vi "emi_Wait for loops to stop.vi"(0 "Loop exlusion[0,..]":u16[](array[numeric])=[0], 7 "Timeout ms(5000)":i32=5000, 11 "error in (no error)":errorcluster) -> (15 "error out":errorcluster)   [LabVIEW 2011]
doc: "Wait for all indexed loops to close. Generates error if times out.\n\nRens regardless of error"
uses:
  Loop control/Private/_emi_Loop control int action.ctl
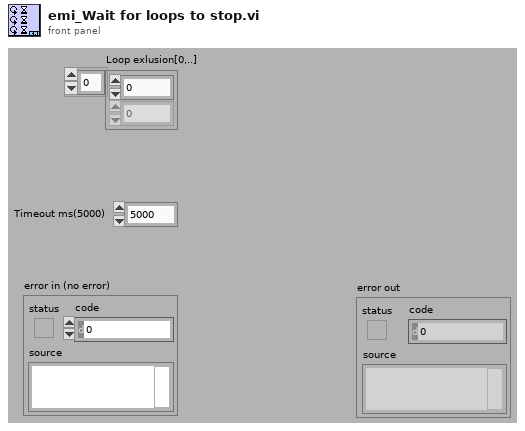
[diagram p1: front panel]
types:
  T1 = typedef "_emi_Loop control int action.ctl" = enum16{"Init index", "Get index", "Set index", "Get Size"}
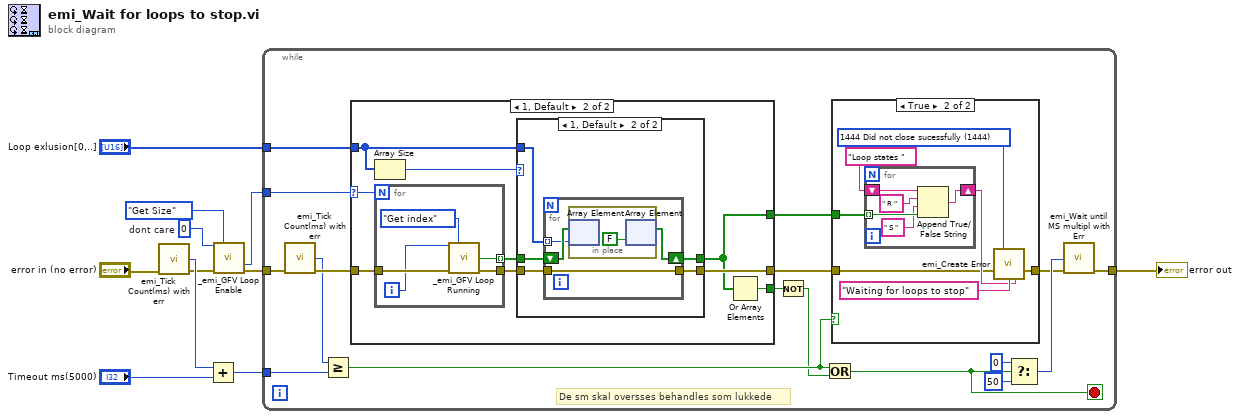
[diagram p0: block diagram]
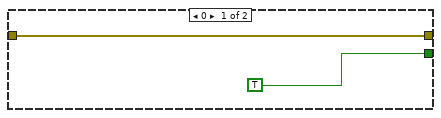
[diagram p3: hidden frame]
diagram:
  w1 = 0  # dont care
  n1 = call "emi_Tick Count(ms) with err.vi"("error in (no error)"="error in (no error)") -> ("millisecond timer value"=w7:u32, "error out"=w5:errorcluster)  [unwired: 13 in]
  n2 = Add(x=w7, y="Timeout ms(5000)") -> (x+y=w2:u32)
  n3 = call "_emi_GFV Loop Enable.vi"("Loop Index/Numb"=w1, "Action(Get Index)"=_emi_Loop_control_int_action."Get Size", "error in (no error)"=w5) -> ("Size"=w3:i32, "error out"=w4:errorcluster)  [unwired: 9 in, 2 out]
  n4 = while {
    tunnel: "Loop exlusion[0,..]" -> [w28]
    tunnel: [w27] -> w10
    tunnel: w4 -> [w22]
    tunnel: w3 -> [w23]
    tunnel: w2 -> [w20]
    stop <- w12 stop-if-true
    # "De sm skal oversses behandles som lukkede"
    n5 = call "emi_Tick Count(ms) with err.vi"("error in (no error)"=w22) -> ("millisecond timer value"=w19:u32, "error out"=w21:errorcluster)  [unwired: 13 in]
    n6 = Greater Or Equal?(x=w19, y=w20) -> (x >= y?=w15:bool)
    n7 = case shown="1, Default" w23 {
      selector: w23 -> [_ w51]
      tunnel: w21 -> [w43 w52]
      tunnel: w28 -> [_ w47]
      tunnel: [w43 w46] -> w18
      tunnel: [TRUE w44] -> w14
      tunnel: [_ w45] -> w17
      frame 0 {
      }
      frame 1, Default {
        n8 = Array Size(array=w47) -> (size(s)=w49:i32)
        n9 = for {
          N: w51 -> [_]
          tunnel: w52 -> [w69]
          tunnel: [w68] -> w50
          tunnel: [w65] -> w48 mode=indexing
          i -> [w66]
          n10 = call "_emi_GFV Loop Running.vi"("Loop Index/Numb"=w66, "Action(Get Index)"=_emi_Loop_control_int_action."Get index", "error in (no error)"=w69) -> ("Loop Running Out"=w65:bool, "error out"=w68:errorcluster)  [unwired: 9 in, 2 out]
        }
        n11 = case shown="1, Default" w49 {
          tunnel: w50 -> [w54 w58]
          tunnel: [w54 w59] -> w46
          tunnel: [w53 w55] -> w45
          tunnel: w48 -> [w53 w56]
          tunnel: w47 -> [_ w57]
          frame 0 {
          }
          frame 1, Default {
            n12 = for {
              tunnel: [w63] -> w59
              tunnel: w58 -> [w63]
              tunnel: w57 -> [w60] mode=indexing
              shift-right: [w61] -> w55
              shift-left: w56 -> [w62]
              n13 = in-place {
                n14 = in-place-array #1(w62, w60) -> ()  [unwired: 1 out]
                n15 = in-place-array #1(FALSE) -> (w61:bool[])  [unwired: 1 out]
              }
            }
          }
        }
        n16 = Or Array Elements(Boolean array=w45) -> (logical OR=w44:bool)
      }
    }
    n17 = Not(x=w14) -> (.not. x?=w13:bool)
    n18 = Or(x=w15, y=w13) -> (x .or. y?=w12:bool)
    n19 = case shown="True" w15 {
      tunnel: [w29 w30] -> w16
      tunnel: w18 -> [w29 w31]
      tunnel: w17 -> [_ w33]
      frame False {
      }
      frame True {
        w35 = 1444 items=["0 No Error"=0, "1 Invalid input parameter"=1, "6 Generic file IO "=6, "7 File not Found"=7, "35 Generic Pring Error"=35, "37 Device not Found"=37, "39 Device Unit Error"=39, "40 Could fot Open Device"=40, "42 Generic Error"=42, "52 Unknown Message"=52, "98 Bad File type"=98, "99 Bad File Version"=99, "100 Bad Data in File"=100, "1018 Unspecefied Error"=1018, "1041 Incorrect Password"=1041, "1043 Feature not in this version"=1043, "1109 Unsuported Data type"=1109, "1444 Did not close sucessfully"=1444] ("Error Code")
        n20 = for {
          shift-right: [w40] -> w32
          shift-left: "Loop states " ("string (\"\")") -> [w41]
          tunnel: w33 -> [w39] mode=indexing
          n21 = Append True/False String(1:w39, 2:" S " ("false string"), 3:" R " ("true string"), 4:w41) -> (0:w40:string)
        }
        n22 = call "emi_Create Error.vi"("Error Code"=w35, "error in (no error)"=w31, "Source String(\"\")"="Waiting for loops to stop" ("Source String(\"\")"), "Append String(\"\")"=w32) -> ("error out"=w30:errorcluster)  [unwired: 11 in]
      }
    }
    n23 = Select(t=u32 0 ("millisecond multiple(0)"), s=w12, f=u32 50 ("millisecond multiple(0)")) -> (s? t:f=w24:u32)
    n24 = call "emi_Wait until MS multipl with Err.vi"("millisecond multiple(0)"=w24, "error in (no error)"=w16) -> ("error out"=w27:errorcluster)  [unwired: 13 in]
  }
  "error out" <- w10
